vi "CRC16.vi"(9 "输入数组":u8[](array[numeric]) format="%.0x", 10 "输入字符串":string, 11 "输入方式":enum16{"数组", "字符串"}(ring)=enum."字符串") -> (1 "CRC16(String)":string, 2 "CRC16":i32 format="%.0x")   [LabVIEW 2015]
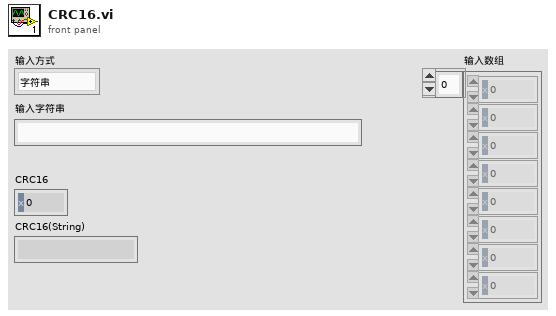
[diagram p1: front panel]
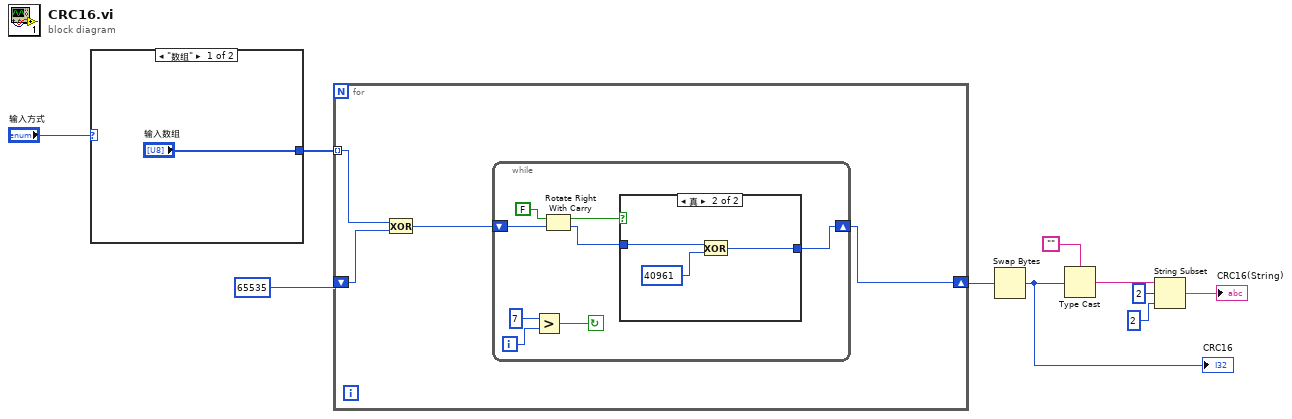
[diagram p0: block diagram]
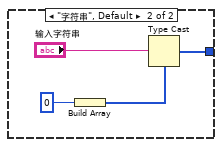
[diagram p2: hidden frame]
diagram:
  n1 = case shown="\"数组\"" "输入方式" {
    tunnel: ["输入数组" w15] -> w10
    frame "数组" {
    }
    frame "字符串", Default {
      n2 = Build Array(u8 0) -> (w13:u8[])
      n3 = Type Cast(type=w13, x="输入字符串") -> (*(type *) &x=w15:u8[])
    }
  }
  n4 = for {
    tunnel: w10 -> [w18] mode=indexing
    shift-right: [w16] -> w8
    shift-left: 65535 -> [w19]
    n5 = Exclusive Or(1:w19, 2:w18) -> (0:w17:i32)
    n6 = while {
      shift-right: [w23] -> w16
      shift-left: w17 -> [w27]
      i -> [w22]
      stop <- w20 continue-if-true
      n7 = Greater?(x=7, y=w22) -> (0:w20:bool)
      n8 = Rotate Right With Carry(2:w27, 3:FALSE) -> (0:w24:i32, 1:w25:bool)
      n9 = case shown="真" w25 {
        tunnel: w24 -> [w28 w31]
        tunnel: [w28 w29] -> w23
        frame False {
        }
        frame True {
          n10 = Exclusive Or(1:40961, 2:w31) -> (0:w29:i32)
        }
      }
    }
  }
  n11 = Swap Bytes(anything=w8) -> (byte swapped=w7:i32)
  "CRC16" <- w7
  n12 = Type Cast(type="", x=w7) -> (*(type *) &x=w6:string)
  n13 = String Subset(string=w6, offset (0)=2 ("偏移量(0)"), length (rest)=2 ("偏移量(0)")) -> (substring=→"CRC16(String)":string)
